vi "SeCrTs-Irms_Module_A.vi"(7 "Data FIFO Ref":T1, 8 "error in":errorcluster, 11 "TCP Network Connection in":refnum<k5>) -> (0 "error out":errorcluster, 3 "TCP Network Connection out":refnum<k5>)   [LabVIEW 2022 SP3]
uses:
  <vilib>/Analysis/3filter.llb/Filter Passband Type.ctl
  <vilib>/Analysis/NI_AALBase.lvlib
  <vilib>/ptbypt/NI_PtbyPt.lvlib
  RT Support/SeCrTs-RT_Global_R.vi
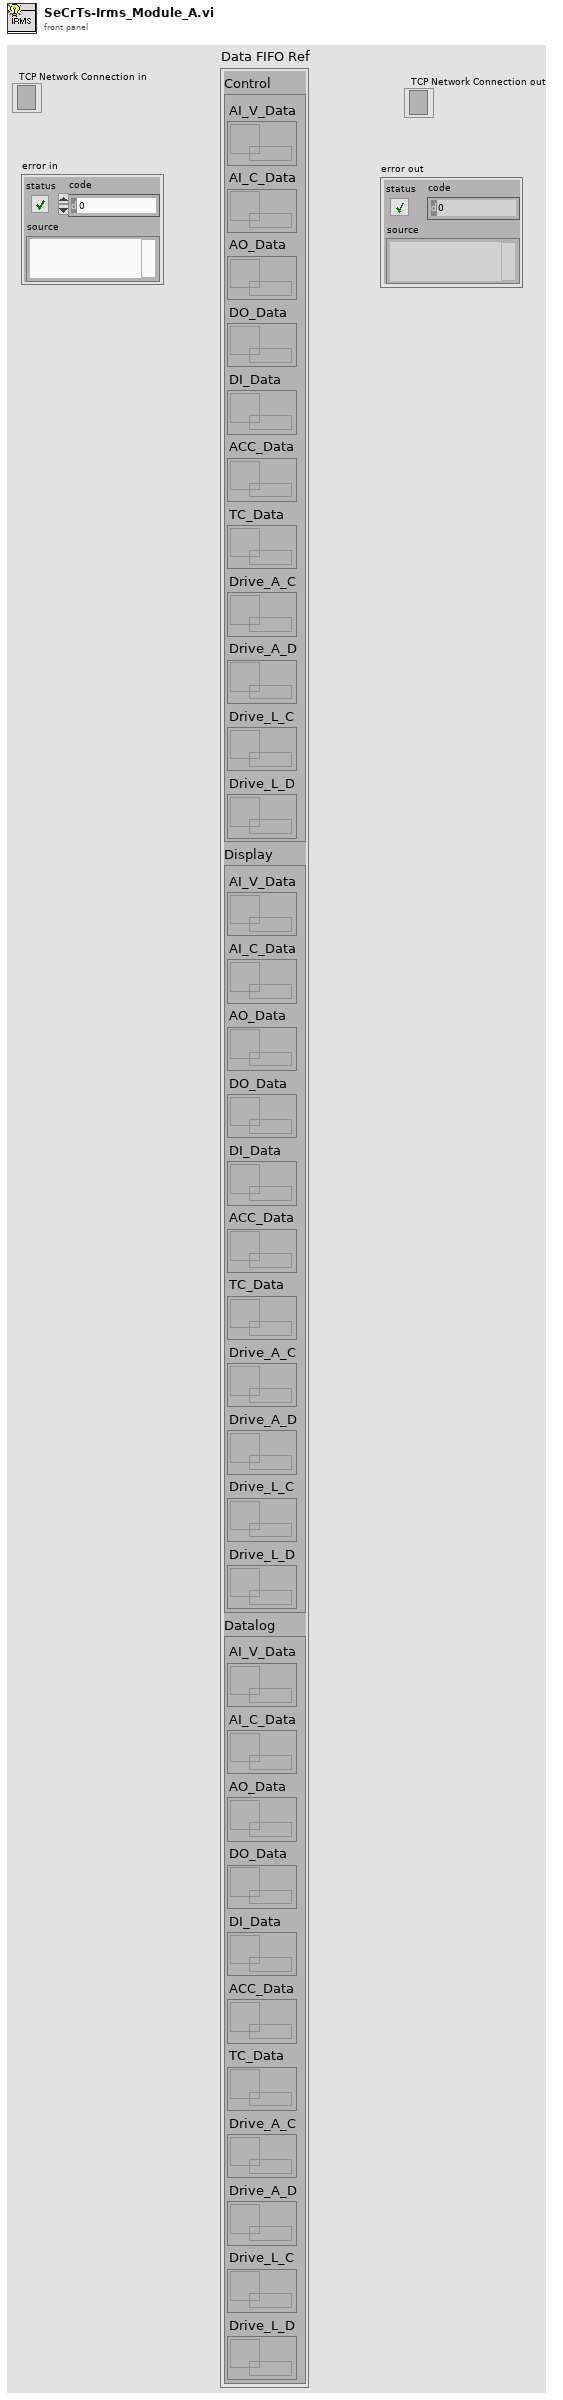
[diagram p1: front panel]
types:
  T1 = cluster{"Control":cluster{"AI_V_Data":refnum<queue>, "AI_C_Data":refnum<queue>, "AO_Data":refnum<queue>, "DO_Data":refnum<queue>, "DI_Data":refnum<queue>, "ACC_Data":refnum<queue>, "TC_Data":refnum<queue>, "Drive_A_C":refnum<queue>, "Drive_A_D":refnum<queue>, "Drive_L_C":refnum<queue>, "Drive_L_D":refnum<queue>}, "Display":cluster{"AI_V_Data":refnum<queue>, "AI_C_Data":refnum<queue>, "AO_Data":refnum<queue>, "DO_Data":refnum<queue>, "DI_Data":refnum<queue>, "ACC_Data":refnum<queue>, "TC_Data":refnum<queue>, "Drive_A_C":refnum<queue>, "Drive_A_D":refnum<queue>, "Drive_L_C":refnum<queue>, "Drive_L_D":refnum<queue>}, "Datalog":cluster{"AI_V_Data":refnum<queue>, "AI_C_Data":refnum<queue>, "AO_Data":refnum<queue>, "DO_Data":refnum<queue>, "DI_Data":refnum<queue>, "ACC_Data":refnum<queue>, "TC_Data":refnum<queue>, "Drive_A_C":refnum<queue>, "Drive_A_D":refnum<queue>, "Drive_L_C":refnum<queue>, "Drive_L_D":refnum<queue>}}
  T2 = typedef "NI_AALBase.lvlib/Filter Passband Type.ctl" = enum32{"Lowpass", "Highpass", "Bandpass", "Bandstop"}
  T3 = cluster{"En_Drive_A":bool, "En_Drive_L":bool, "Exit_Drive_A":bool, "Exit_Drive_L":bool}
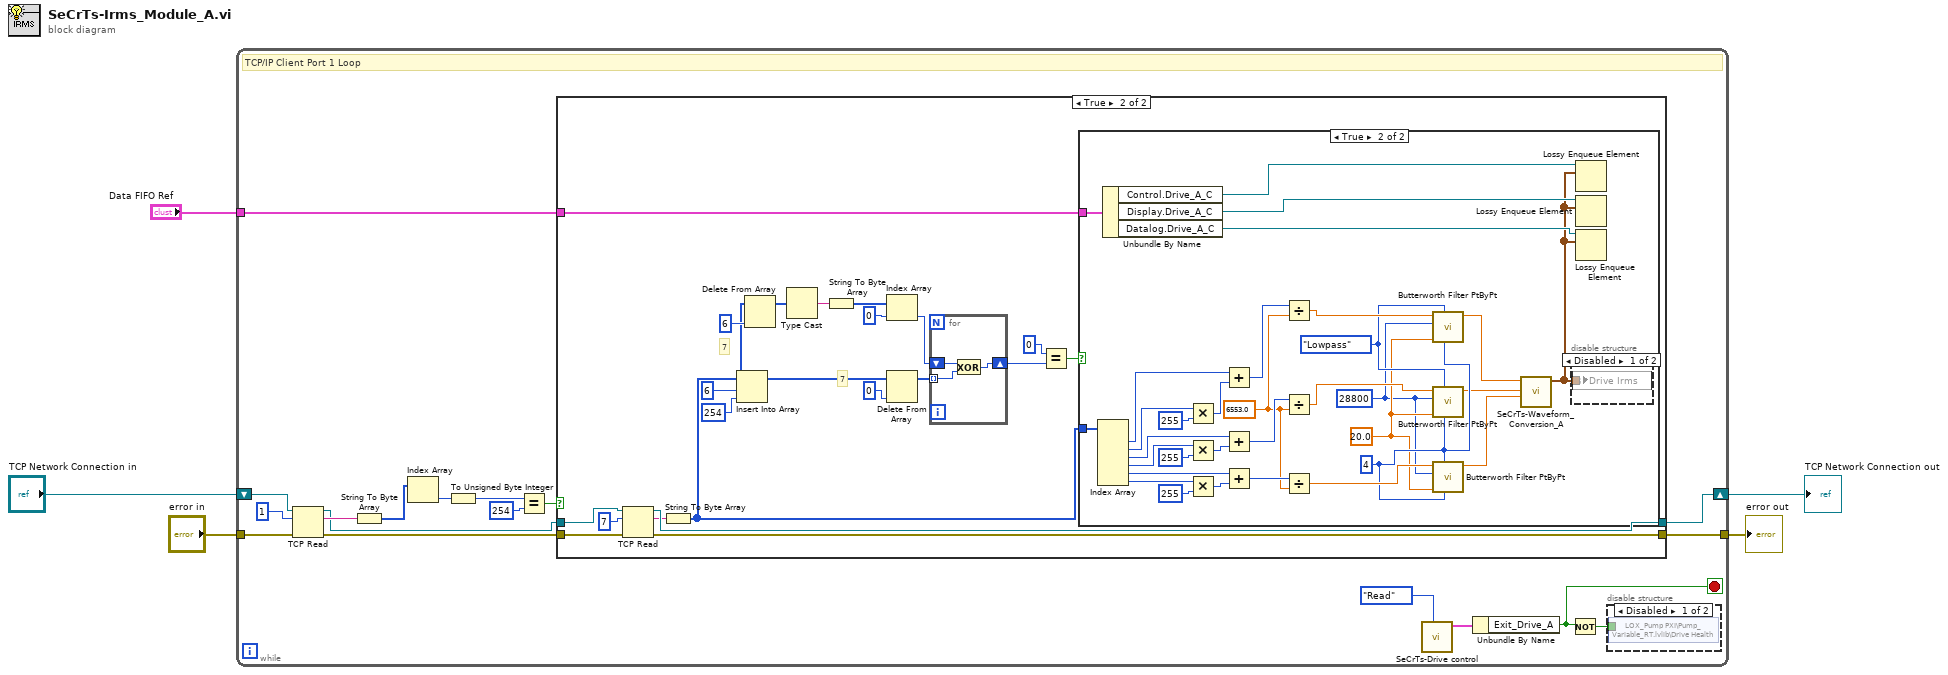
[diagram p0: block diagram]
diagram:
  n1 = while {
    tunnel: [w15] -> w3
    shift-right: [w14] -> w4
    shift-left: "TCP Network Connection in" -> [w23]
    tunnel: "error in" -> [w11]
    tunnel: "Data FIFO Ref" -> [w6]
    stop <- w8 stop-if-true
    # "TCP/IP Client Port 1 Loop"
    n2 = TCP Read(connection ID=w23, bytes to read=1, error in (no error)=w11) -> (connection ID out=w16:refnum<k5>, data out=w17:string, error out=w12:errorcluster)  [unwired: 2 in]
    n3 = String To Byte Array(string=w17) -> (unsigned byte array=w21:u8[])
    n4 = Index Array(array=w21) -> (element=w20:u8)  [unwired: 1 in]
    n5 = To Unsigned Byte Integer(number=w20) -> (unsigned 8bit integer=w19:u8)
    n6 = Equal?(x=w19, y=u8 254) -> (x = y?=w13:bool)
    n7 = case shown="True" w13 {
      tunnel: w16 -> [w25 w48]
      tunnel: w12 -> [w26 w47]
      tunnel: [w26 w46] -> w15
      tunnel: [w25 w45] -> w14
      tunnel: w6 -> [_ w27]
      frame False {
      }
      frame True {
        # "7"
        # "7"
        n8 = TCP Read(connection ID=w48, bytes to read=7, error in (no error)=w47) -> (connection ID out=w45:refnum<k5>, data out=w44:string, error out=w46:errorcluster)  [unwired: 2 in]
        n9 = String To Byte Array(string=w44) -> (unsigned byte array=w31:u8[])
        n10 = Insert Into Array(array=w31, index=6, new element=u8 254 ("new element/subarray")) -> (w32:u8[])
        n11 = Delete From Array(array=w31, index=6) -> (array with subset deleted=w35:u8[])  [unwired: 1 in, 1 out]
        n12 = Type Cast(x=w35) -> (*(type *) &x=w41:string)  [unwired: 1 in]
        n13 = String To Byte Array(string=w41) -> (unsigned byte array=w36:u8[])
        n14 = Index Array(array=w36, index=0) -> (element=w39:u8)
        n15 = Delete From Array(array=w32, index=0) -> (array with subset deleted=w38:u8[])  [unwired: 1 in, 1 out]
        n16 = for {
          shift-right: [w83] -> w29
          shift-left: w39 -> [w84]
          tunnel: w38 -> [w82] mode=indexing
          n17 = Exclusive Or(1:w82, 2:w84) -> (0:w83:u8)
        }
        n18 = Equal?(x=u8 0, y=w29) -> (x = y?=w28:bool)
        n19 = case shown="True" w28 {
          tunnel: w31 -> [_ w65]
          tunnel: w27 -> [_ w53]
          frame False {
          }
          frame True {
            w60 = Filter_Passband_Type."Lowpass" ("filter type")
            w59 = 4 ("order")
            w58 = 20.0 ("low cutoff freq: fl")
            w57 = 28800 ("rank")
            w64 = 6553.0
            n20 = Index Array(array=w65) -> (element #1=w78:u8, element #2=w77:u8, element #3=w72:u8, element #4=w71:u8, element #5=w70:u8, element #6=w69:u8)  [unwired: 6 in]
            n21 = Unbundle By Name(w53) -> ("Control.Drive_A_C"=w52:refnum<queue>, "Display.Drive_A_C"=w51:refnum<queue>, "Datalog.Drive_A_C"=w50:refnum<queue>)
            n22 = Multiply(x=w77, y=u32 255) -> (x*y=w79:u32)
            n23 = Multiply(x=w71, y=u32 255) -> (x*y=w76:u32)
            n24 = Multiply(x=w69, y=u32 255) -> (x*y=w73:u32)
            n25 = Add(x=w78, y=w79) -> (x+y=w68:u32)
            n26 = Add(x=w72, y=w76) -> (x+y=w67:u32)
            n27 = Add(x=w70, y=w73) -> (x+y=w66:u32)
            n28 = Divide(x=w68, y=w64) -> (x/y=w63:dbl)
            n29 = Divide(x=w67, y=w64) -> (x/y=w62:dbl)
            n30 = Divide(x=w66, y=w64) -> (x/y=w61:dbl)
            n31 = call <vilib>:"Butterworth Filter PtByPt.vi"("order"=w59, "filter type"=w60, "low cutoff freq: fl"=w58, "sampling freq: fs"=w57, "x"=w63) -> ("Filtered x"=w56:dbl)  [unwired: 4 in, 1 out]
            n32 = call <vilib>:"Butterworth Filter PtByPt.vi"("order"=w59, "filter type"=w60, "low cutoff freq: fl"=w58, "sampling freq: fs"=w57, "x"=w62) -> ("Filtered x"=w55:dbl)  [unwired: 4 in, 1 out]
            n33 = call <vilib>:"Butterworth Filter PtByPt.vi"("order"=w59, "filter type"=w60, "low cutoff freq: fl"=w58, "sampling freq: fs"=w57, "x"=w61) -> ("Filtered x"=w54:dbl)  [unwired: 4 in, 1 out]
            n34 = call "SeCrTs-Waveform_Conversion_A.vi"("Irms3"=w54, "Irms2"=w55, "Irms1"=w56) -> ("Array"=w49:waveform(dbl)[])  [unwired: 8 in]
            n35 = disable-structure shown="Disabled" {
              disable-tunnel: w49 -> [w81 _]
              frame Disabled {
                n36 = global write "SeCrTs-RT_Global_R.vi" "Drive Irms"(w81) -> ()
              }
              frame Enabled {
              }
            }
            n37 = Lossy Enqueue Element(queue=w52, element=w49) -> ()  [unwired: 1 in, 4 out]
            n38 = Lossy Enqueue Element(queue=w51, element=w49) -> ()  [unwired: 1 in, 4 out]
            n39 = Lossy Enqueue Element(queue=w50, element=w49) -> ()  [unwired: 1 in, 4 out]
          }
        }
      }
    }
    n40 = call "SeCrTs-Drive control.vi"("Action"=enum16{"Init", "Write", "Read"}."Read") -> ("Loop Control Out"=w9:T3)  [unwired: 9 in, 1 out]
    n41 = Unbundle By Name(w9) -> ("Exit_Drive_A"=w8:bool)
    n42 = Not(x=w8) -> (.not. x?=w10:bool)
    n43 = disable-structure shown="Disabled" {
      disable-tunnel: w10 -> [w24 _]
      frame Disabled {
        n44 = shared-variable "LOX_Pump PXI\\Pump_Variable_RT.lvlib\\Drive Health"(w24) -> ()  [unwired: 1 in, 1 out]
      }
      frame Enabled {
      }
    }
  }
  "TCP Network Connection out" <- w4
  "error out" <- w3
